vi "DESRound.vi"(2 "SubKey":bool[](array[boolean]), 3 "Left":bool[](array[boolean]), 5 "Right":bool[](array[boolean])) -> (0 "NewLeft":bool[](array[boolean]), 1 "NewRight":bool[](array[boolean]))   [LabVIEW 2013]
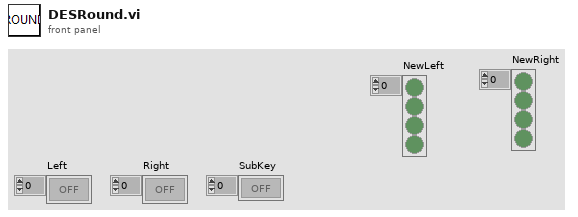
[diagram p1: front panel]
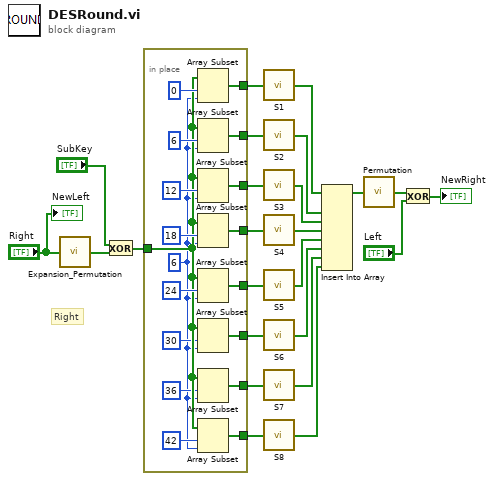
[diagram p0: block diagram]
diagram:
  # "Right"
  n1 = call "Expansion_Permutation.vi"("array"="Right") -> ("Array"=w24:bool[])
  n2 = Exclusive Or(1:w24, 2:"SubKey") -> (0:w9:bool[])
  n3 = in-place {
    in-place-border: w9 -> [w37]
    in-place-border: [w32] -> w8
    in-place-border: [w31] -> w7
    in-place-border: [w30] -> w6
    in-place-border: [w29] -> w5
    in-place-border: [w28] -> w4
    in-place-border: [w27] -> w3
    in-place-border: [w26] -> w2
    in-place-border: [w25] -> w1
    w33 = 6 ("length")
    n4 = Array Subset(array=w37, index=0, length=w33) -> (w32:bool[])
    n5 = Array Subset(array=w37, index=6, length=w33) -> (w31:bool[])
    n6 = Array Subset(array=w37, index=12, length=w33) -> (w30:bool[])
    n7 = Array Subset(array=w37, index=18, length=w33) -> (w29:bool[])
    n8 = Array Subset(array=w37, index=24, length=w33) -> (w28:bool[])
    n9 = Array Subset(array=w37, index=30 ("length"), length=w33) -> (w27:bool[])
    n10 = Array Subset(array=w37, index=36, length=w33) -> (w26:bool[])
    n11 = Array Subset(array=w37, index=42, length=w33) -> (w25:bool[])
  }
  n12 = call "S1.vi"("Input array"=w8) -> ("Array"=w23:bool[])
  n13 = call "S2.vi"("Input array"=w7) -> ("Array"=w22:bool[])
  n14 = call "S3.vi"("Input array"=w6) -> ("Array"=w21:bool[])
  n15 = call "S4.vi"("Input array"=w5) -> ("Array"=w20:bool[])
  n16 = call "S5.vi"("Input array"=w4) -> ("Array"=w19:bool[])
  n17 = call "S6.vi"("Input array"=w3) -> ("Array"=w18:bool[])
  n18 = call "S7.vi"("Input array"=w2) -> ("Array"=w17:bool[])
  n19 = call "S8.vi"("Input array"=w1) -> ("Array"=w16:bool[])
  n20 = Insert Into Array(array=w23, new element #1=w22, new element #2=w21, new element #3=w20, new element #4=w19, new element #5=w18, new element #6=w17, new element #7=w16) -> (w10:bool[])  [unwired: 1 in]
  n21 = call "Permutation.vi"("array"=w10) -> ("Array"=w12:bool[])
  n22 = Exclusive Or(1:"Left", 2:w12) -> (0:→"NewRight":bool[])
  "NewLeft" <- "Right"
